vi "dmc_test.vi"() -> ()   [LabVIEW 2018]
uses:
  <vilib>/Utility/miscctls.llb/LVForegroundBackgroundColorsTypeDef.ctl
panel:
  in  "Customizable Tab":enum32{"Page 1", "Page 3"}(tab)
  in  "Preferences Button":bool
  in  "Start Button":bool
  in  "Boolean Switch":bool
  in  "Horizontal Multi-Slider Control":cluster{"Fill":dbl, "Fill":dbl}(slide)={"Fill"=1.0, "Fill"=8.628318584070797} scale=0.0..200000.0
  in  "Numeric Control":dbl
  in  "Listbox":i32(listbox)
  in  "VISA":refnum<visa-resource-name>
  in  "Radio Buttons - Customizable":T1(radio)
  in  "Enum - Menu":enum16{""}(ring)
  out "Waveform Chart - Dark":dbl(graph) caption="Waveform Chart - dark"
  out "2D Picture":picture
  out "Gauge":dbl(knob) scale=0.0..100000.0
  in  "stop":bool
  in  "Preferences Button 2":bool
  in  "Start Button 2":bool
  in  "Boolean Switch 2":bool
  in  "Horizontal Multi-Slider Control 2":cluster{"Fill":dbl, "Fill":dbl}(slide)={"Fill"=1.0, "Fill"=8.628318584070797} scale=0.0..200000.0
  in  "Numeric Control 2":dbl
  in  "Listbox 2":i32(listbox)
  in  "VISA 2":refnum<visa-resource-name>
  in  "Radio Buttons - Customizable 2":T1(radio)
  in  "Enum - Menu 2":enum16{""}(ring)
  out "Waveform Chart - Dark 2":dbl(graph) caption="Waveform Chart - dark"
  out "2D Picture 2":picture
  out "Gauge 2":dbl(knob) caption="Gauge" scale=0.0..100000.0
  in  "stop 2":bool
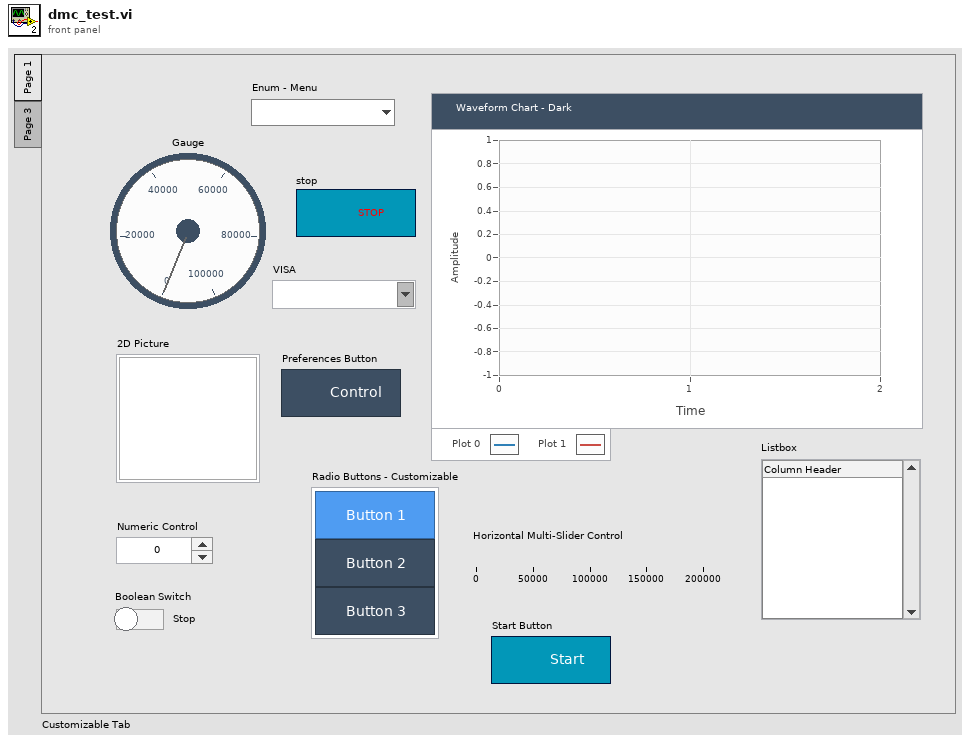
[diagram p1: front panel]
types:
  T1 = enum32{"Standard Button", "Standard Button 2", "Standard Button 3"}
  T2 = typedef "LVForegroundBackgroundColorsTypeDef.ctl" = cluster{"Foreground Color":u32, "Background Color":u32}
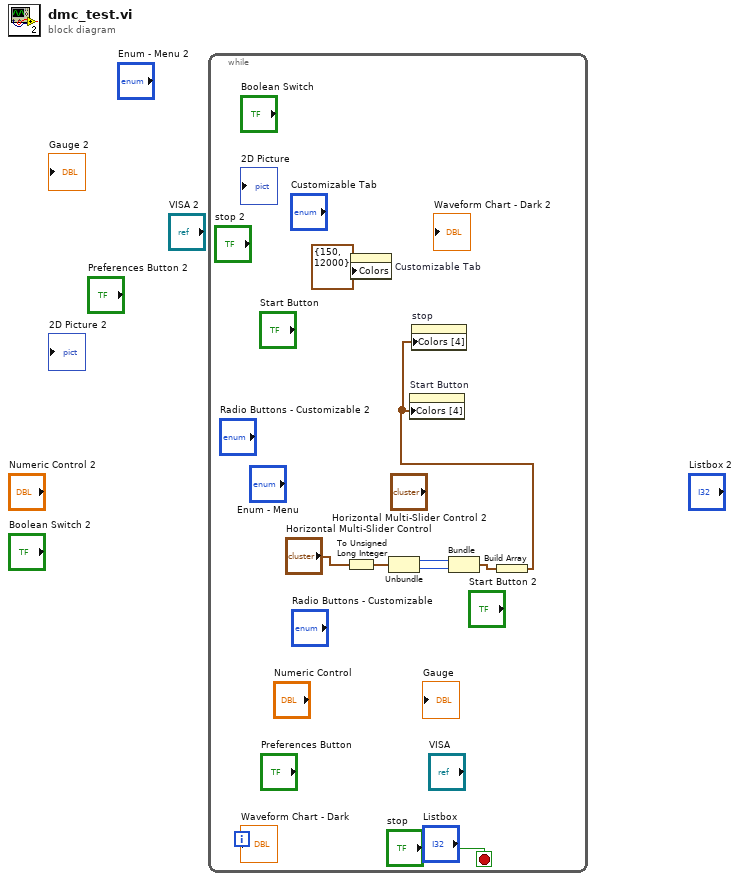
[diagram p0: block diagram]
diagram:
  n1 = while {
    stop <- "stop" stop-if-true
    n2 = To Unsigned Long Integer(number="Horizontal Multi-Slider Control") -> (unsigned 32bit integer=w6:cluster{"Fill":u32, "Fill":u32})
    n3 = property on="Customizable Tab" class="TabCtl (strict)"("Colors"=T2 {"Foreground Color"=150, "Background Color"=12000}) -> ()  [unwired: 2 in, 2 out]
    n4 = Unbundle(w6) -> ("Fill"=w5:u32, "Fill"=w4:u32)
    n5 = Bundle("Fill"=w5, "Fill"=w4) -> (w3:cluster{"Fill":u32, "Fill":u32})  [unwired: 1 in]
    n6 = Build Array(w3) -> (w2:cluster{"Fill":u32, "Fill":u32}[])
    n7 = property on="Start Button" class="Bool"("Colors [4]"=w2) -> ()  [unwired: 2 in, 2 out]
    n8 = property on="stop" class="Bool"("Colors [4]"=w2) -> ()  [unwired: 2 in, 2 out]
  }
